vi "Main.vi"() -> ()   [LabVIEW 2013]
uses:
  tags_cluster.ctl
  imagereconstruction/x64/Debug/labviewdll.dll
panel:
  out "tiff pointer":i64 format="%x"
  in  "Tab Control":enum32{"Sinograph", "Backprojection"}(tab)
  in  "Contrast with forward proj":bool
  in  "Centre":i32[](array[numeric])
  in  "All slices":bool
  out "Current Slice":i32
  out "Angles":dbl[](array[numeric])
  in  "Number of projections":u32
  in  "slice":u32
  out "Image Properties":T1
  in  "Go":bool
  out "error":i32
  out "Error Out":errorcluster
  out "pixels":u8[](array[numeric])
  in  "Image Number":u32=100
  out "libTIFF Version String":string
  out "Number of Rows":u32
  out "Number of Angles":u32
  in  "Quit":bool
  in  "Data TIFF File":path
  in  "Angle CSV File":path
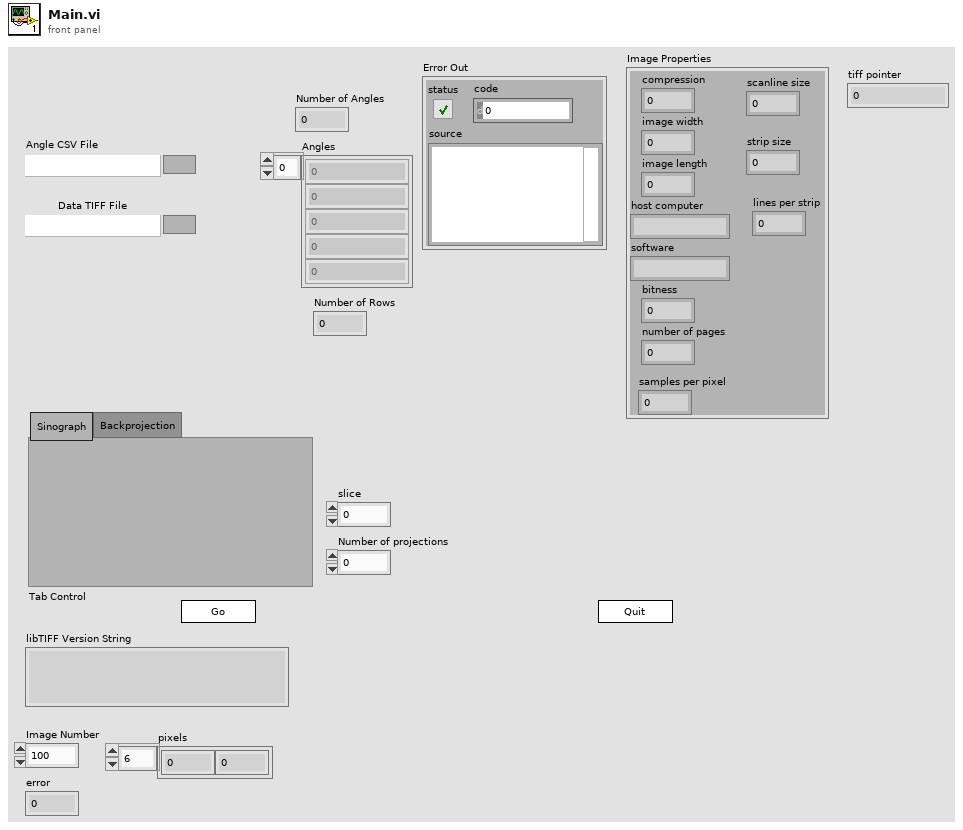
[diagram p1: front panel]
types:
  T1 = typedef "tags_cluster.ctl" = cluster{"compression":i32, "image width":i32, "image length":i32, "host computer":string, "software":string, "bitness":i32, "number of pages":i32, "samples per pixel":i32, "scanline size":i32, "strip size":i32, "lines per strip":i32}
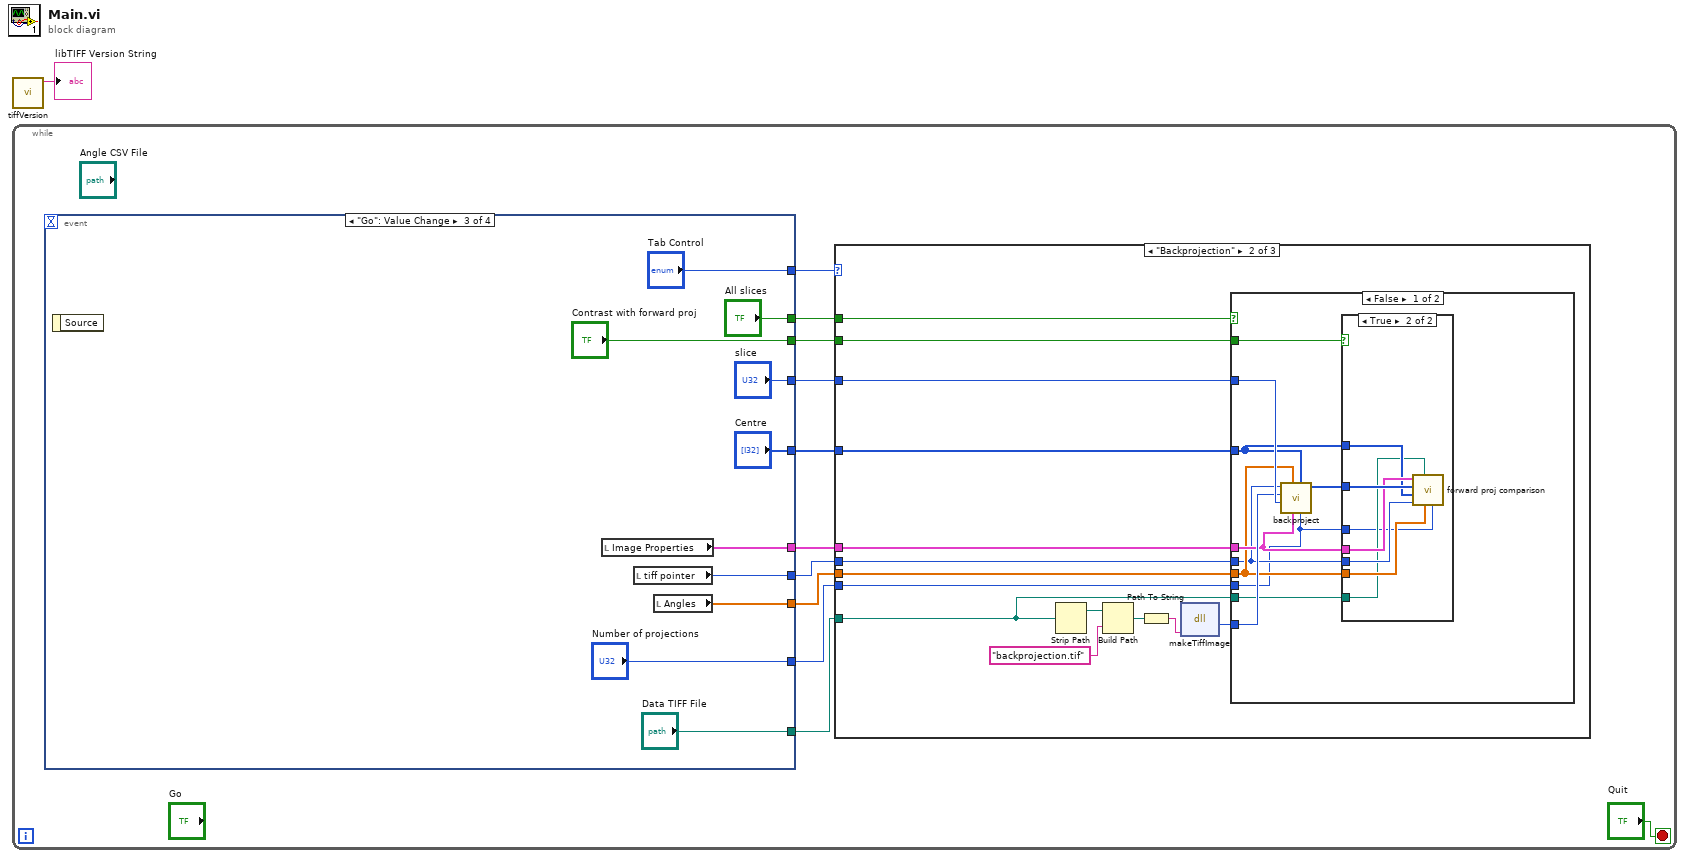
[diagram p0: block diagram]
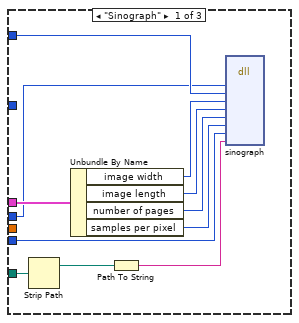
[diagram p2: hidden frame]
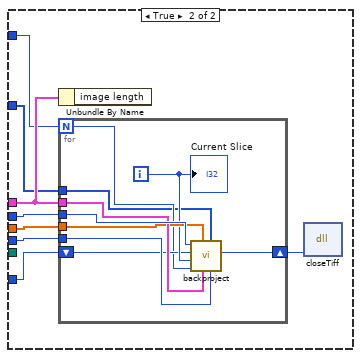
[diagram p4: hidden frame]
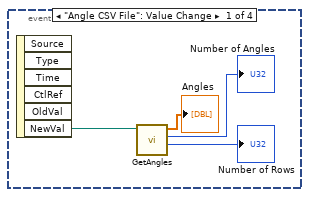
[diagram p6: hidden frame]
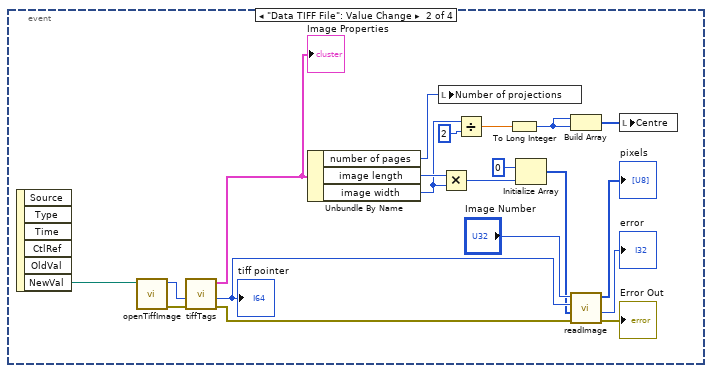
[diagram p7: hidden frame]
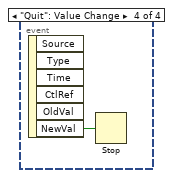
[diagram p8: hidden frame]
diagram:
  n1 = call "tiffVersion.vi"() -> ("tiff_ver"=→"libTIFF Version String":string)  [unwired: 11 in]
  n2 = while {
    stop <- "Quit" stop-if-true
    n3 = event shown="[2] \"Go\": Value Change" {
      selector: _ -> [_ _ _ _]
      dyn-events: _ -> [_ _ _ _]
      timeout: _ -> [_ _ _ _]
      tunnel: [_ _ w105 _] -> w11
      tunnel: [_ _ "slice" _] -> w10
      tunnel: [_ _ "Data TIFF File" _] -> w9
      tunnel: [_ _ w102 _] -> w8
      tunnel: [_ _ w101 _] -> w7
      tunnel: [_ _ "All slices" _] -> w6
      tunnel: [_ _ "Number of projections" _] -> w5
      tunnel: [_ _ "Tab Control" _] -> w4
      tunnel: [_ _ "Centre" _] -> w3
      tunnel: [_ _ "Contrast with forward proj" _] -> w2
      event "Angle CSV File": Value Change {
        n4 = event-data() -> ("NewVal"=w74:path)  [unwired: 1 in, 5 out]
        n5 = call "GetAngles.vi"("NewVal"=w74) -> ("Number of Rows"=→"Number of Rows":u16, "Number of Angles"=→"Number of Angles":i32, "Array"=→"Angles":dbl[])  [unwired: 8 in]
      }
      event "Data TIFF File": Value Change {
        n6 = event-data() -> ("NewVal"=w95:path)  [unwired: 1 in, 5 out]
        n7 = call "openTiffImage.vi"("NewVal"=w95) -> ("error out"=w85:errorcluster, "returned pointer"=w84:i64)  [unwired: 9 in]
        n8 = call "tiffTags.vi"("error in (no error)"=w85, "tif pointer"=w84) -> ("error out"=w91:errorcluster, "tiff pointer"=w92:i64, "Image Properties"=w83:T1)  [unwired: 7 in]
        "Image Properties" <- w83
        "tiff pointer" <- w92
        n9 = Unbundle By Name(w83) -> ("number of pages"=w82:i32, "image length"=w81:i32, "image width"=w79:i32)
        n10 = local write "Number of projections"(w82) -> ()
        n11 = Multiply(x=w81, y=w79) -> (x*y=w86:i32)
        n12 = Divide(x=w79, y=2) -> (x/y=w76:dbl)
        n13 = To Long Integer(number=w76) -> (32bit integer=w77:i32)
        n14 = Initialize Array(u8 0, w86) -> (w88:u8[])
        n15 = Build Array(w77, w77) -> (w80:i32[])
        n16 = call "readImage.vi"("Error in"=w91, "raster"=w88, "tif"=w92, "Image Number"="Image Number") -> ("Error Out"=→"Error Out":errorcluster, "error"=→"error":i32, "pixels"=→"pixels":u8[])  [unwired: 4 in, 1 out]
        n17 = local write "Centre"(w80) -> ()
      }
      event "Go": Value Change {
        n18 = event-data() -> ()  [unwired: 1 in, 1 out]
        n19 = local read "Image Properties"() -> (w101:T1)
        n20 = local read "tiff pointer"() -> (w102:i64)
        n21 = local read "Angles"() -> (w105:dbl[])
      }
      event "Quit": Value Change {
        n22 = event-data() -> ("NewVal"=w106:bool)  [unwired: 1 in, 5 out]
        n23 = Stop(stop? (T)=w106) -> ()
      }
    }
    n24 = case shown="\"Backprojection\"" w4 {
      tunnel: w7 -> [w17 w30 _]
      tunnel: w10 -> [w16 w27 _]
      tunnel: w8 -> [w15 w37 _]
      tunnel: w5 -> [w14 w36 _]
      tunnel: w9 -> [w13 w24 _]
      tunnel: w11 -> [_ w35 _]
      tunnel: w6 -> [_ w34 _]
      tunnel: w3 -> [_ w26 _]
      tunnel: w2 -> [_ w25 _]
      frame "Sinograph" {
        n25 = Strip Path(path=w13) -> (stripped path=w20:path)  [unwired: 1 out]
        n26 = Unbundle By Name(w17) -> ("image width"=w21:i32, "image length"=w23:i32, "number of pages"=w22:i32, "samples per pixel"=w18:i32)
        n27 = Path To String(path=w20) -> (string=w19:string)
        n28 = dll-call lib="D:/work/uni/FYP/reconrepo/imagereconstruction/x64/Debug/labviewdll.dll" fn="sinograph"("tiff pointer"=w15, "slice"=w16, "imageWidth"=w21, "imageLength"=w23, "total_quantity"=w22, "samples_per_pixel"=w18, "used_quantity"=w14, "resultPath"=w19) -> ()  [unwired: 12 in, 2 out]
      }
      frame "Backprojection" {
        n29 = Strip Path(path=w24) -> (stripped path=w33:path)  [unwired: 1 out]
        n30 = Build Path(base path=w33, name or relative path="backprojection.tif") -> (appended path=w32:path)
        n31 = Path To String(path=w32) -> (string=w29:string)
        n32 = dll-call lib="D:/work/uni/FYP/reconrepo/imagereconstruction/x64/Debug/labviewdll.dll" fn="makeTiffImage"("resultPath"=w29) -> ("return type"=w28:i64)  [unwired: 4 in, 2 out]
        n33 = case shown="False" w34 {
          tunnel: w37 -> [w40 w62]
          tunnel: w30 -> [w44 w59]
          tunnel: w27 -> [w47 w56]
          tunnel: w36 -> [w38 w61]
          tunnel: w35 -> [w43 w60]
          tunnel: w28 -> [w46 w58]
          tunnel: w26 -> [w42 w55]
          tunnel: w25 -> [w41 _]
          tunnel: w24 -> [w39 _]
          frame False {
            n34 = call "backproject.vi"("Number of projections"=w38, "Centre"=w42, "Image Properties"=w44, "Angles"=w43, "slice"=w47, "output tiff pointer"=w46, "tiff pointer"=w40) -> ("Output"=w45:u8[])  [unwired: 3 in, 1 out]
            n35 = case shown="True" w41 {
              tunnel: w45 -> [_ w54]
              tunnel: w44 -> [_ w53]
              tunnel: w43 -> [_ w52]
              tunnel: w42 -> [_ w51]
              tunnel: w40 -> [_ w50]
              tunnel: w39 -> [_ w49]
              tunnel: w38 -> [_ w48]
              frame False {
              }
              frame True {
                n36 = call "forward proj comparison.vi"("number of projections"=w48, "Angles"=w52, "path name"=w49, "source tiff pointer"=w50, "Centre"=w51, "Output"=w54, "Image Properties"=w53) -> ()  [unwired: 5 in]
              }
            }
          }
          frame True {
            n37 = Unbundle By Name(w59) -> ()  [unwired: 1 out]
            n38 = for {
              N: w56 -> [w64]
              tunnel: w62 -> [w71]
              tunnel: w59 -> [w70]
              tunnel: w61 -> [w69]
              tunnel: w60 -> [w68]
              shift-right: [w65] -> w57
              shift-left: w58 -> [w66]
              tunnel: w55 -> [w63]
              i -> [w67]
              n39 = call "backproject.vi"("Number of projections"=w69, "Centre"=w63, "Image Properties"=w70, "Angles"=w68, "number of pages"=w64, "slice"=w67, "output tiff pointer"=w66, "tiff pointer"=w71) -> ("result tif"=w65:i64)  [unwired: 2 in, 1 out]
              "Current Slice" <- w67
            }
            n40 = dll-call lib="D:/work/uni/FYP/reconrepo/imagereconstruction/x64/Debug/labviewdll.dll" fn="closeTiff"("tiff"=w57) -> ()  [unwired: 5 in, 2 out]
          }
        }
      }
      frame Default {
      }
    }
  }
